vi "LogToDashboard.vi"(3 "error in (no error)":errorcluster, 4 "Info":string) -> (0 "error out":errorcluster)   [LabVIEW 2012]
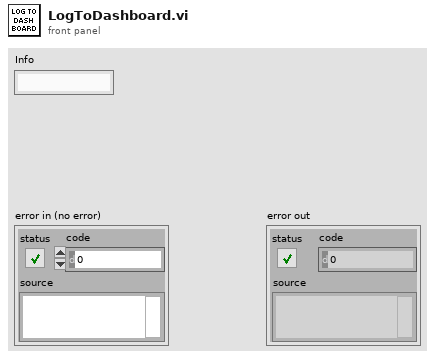
[diagram p1: front panel]
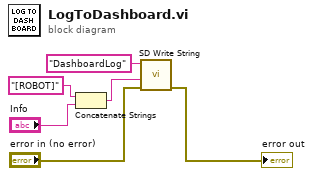
[diagram p0: block diagram]
diagram:
  n1 = Concatenate Strings("[ROBOT]" ("string"), "Info") -> (w3:string)
  n2 = call <vilib>:"SD Write String.vi"("error in"="error in (no error)", "String"=w3, "Name"="DashboardLog") -> ("error out"=→"error out":errorcluster)  [unwired: 7 in, 1 out]
